vi "Draw Text.vi"(8 "error in (no error)":errorcluster, 11 "Terminal in":refnum<class "Terminal.lvclass">) -> (0 "error out":errorcluster, 3 "Terminal out":refnum<class "Terminal.lvclass">)   [LabVIEW 2020, in "Terminal.lvlib" / "Terminal.lvclass"]
uses:
  Terminal.lvclass
  Text Attributes.ctl
  Terminal.lvclass/Terminal.ctl
  TermBuffer/TermBuffer.lvclass
  Terminal.lvlib
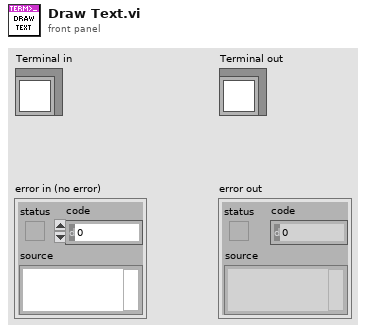
[diagram p1: front panel]
types:
  T1 = cluster{"left":i16, "top":i16, "right":i16, "bottom":i16}
  T2 = enum16{"User-specified Font", "Application Font", "System Font", "Dialog Font"}
  T3 = typedef "Terminal.lvlib/Text Attributes.ctl" = cluster{"FG":u32, "BG":u32, "Bold":bool, "Italic":bool, "Underline":bool, "Strike":bool, "Inverse":bool}
  T4 = typedef "Terminal.lvlib/Terminal.lvclass/Ref Data.ctl" = cluster{"Connection":refnum<class "Connection.lvclass">, "Read Loop Running":bool, "Parse State":T5, "Terminal Options":T9, "Font Metrics":T12}
  T5 = typedef "Terminal.lvlib/Terminal.lvclass/Parse State.ctl" = cluster{"Buffer State":T6, "Cursor":T7, "Attributes":T3}
  T6 = typedef "Terminal.lvlib/Terminal.lvclass/Buffer State.ctl" = cluster{"Sequence":string, "ESC":bool, "Alt Buf":bool}
  T7 = typedef "Terminal.lvlib/Terminal.lvclass/Cursor.ctl" = cluster{"Cur":T8, "Saved":T8}
  T8 = typedef "Terminal.lvlib/Terminal.lvclass/Position.ctl" = cluster{"Row":i32, "Col":i32}
  T9 = typedef "Terminal.lvlib/Terminal Options.ctl" = cluster{"Implied CR with LF":bool, "Local Echo":bool, "Tab Width":i32, "Color Scheme":T10, "Default FG":T11, "Default BG":T11, "History Length":i32, "Font Face":string, "Font Size":i16, "Rows":i32, "Cols":i32}
  T10 = typedef "Terminal.lvlib/Color Scheme.ctl" = cluster{"Black":u32, "Red":u32, "Green":u32, "Yellow":u32, "Blue":u32, "Magenta":u32, "Cyan":u32, "White":u32, "Bright Black":u32, "Bright Red":u32, "Bright Green":u32, "Bright Yellow":u32, "Bright Blue":u32, "Bright Magenta":u32, "Bright Cyan":u32, "Bright White":u32}
  T11 = typedef "Terminal.lvlib/Color.ctl" = i8
  T12 = typedef "Terminal.lvlib/Terminal.lvclass/Font Metrics.ctl" = cluster{"Width":i16, "Height":i16}
  T13 = typedef "Terminal.lvlib/Term Char.ctl" = cluster{"Char":string, "Attributes":T3}
  T14 = cluster{"Font Name:":string, "Size":i16, "Strikeout?":bool, "Italic?":bool, "Underline?":bool, "Outline?":bool, "Shadow?":bool, "Bold?":bool}
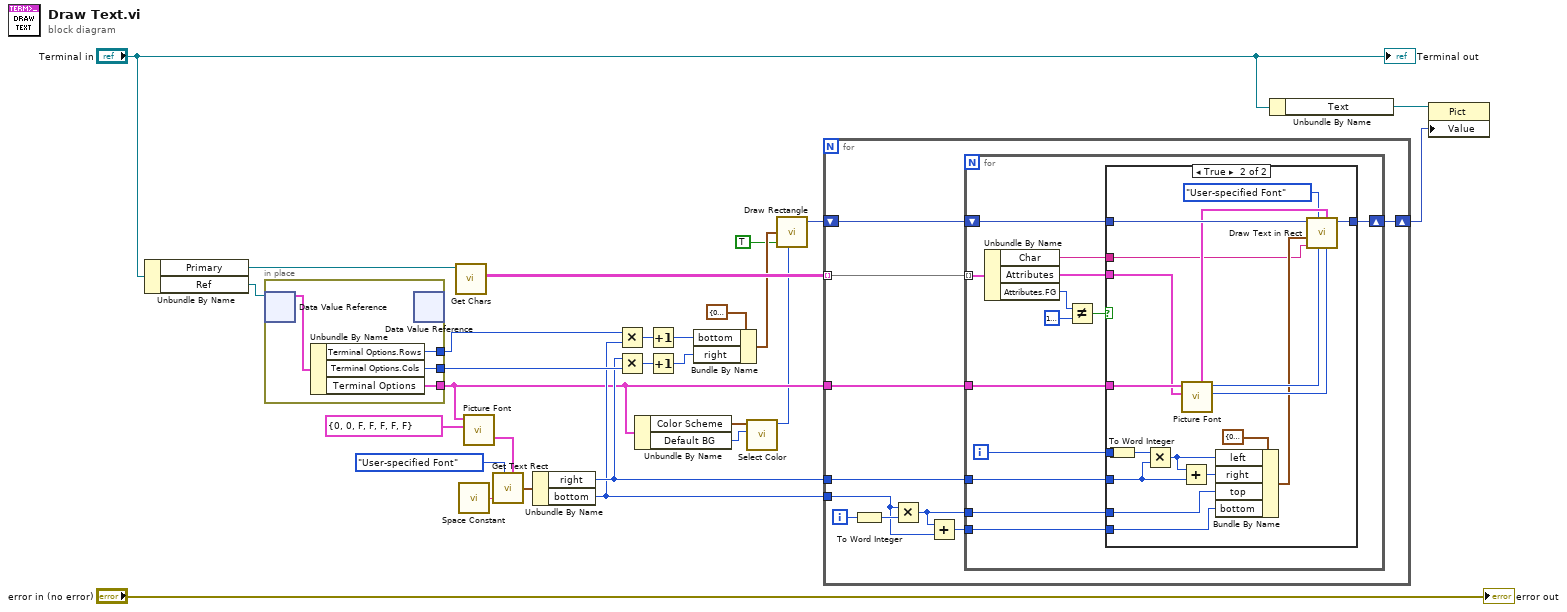
[diagram p0: block diagram]
diagram:
  n1 = Unbundle By Name("Terminal in") -> ("Primary"=w27:refnum<class "TermBuffer.lvclass">, "Ref"=w25:refnum<data-value>)
  n2 = in-place {
    in-place-border: [w31] -> w6
    in-place-border: [w30] -> w13
    in-place-border: [w29] -> w9
    n3 = in-place-dvr #1(w25) -> (w32:T4)  [unwired: 1 out]
    n4 = Unbundle By Name(w32) -> ("Terminal Options.Rows"=w29:i32, "Terminal Options.Cols"=w30:i32, "Terminal Options"=w31:T9)
    n5 = in-place-dvr #1() -> ()  [unwired: 1 in, 2 out]
  }
  n6 = call "Get Chars.vi"("TermBuffer in"=w27) -> ("TermChars"=w26:T13[][])  [unwired: 8 in, 2 out]
  n7 = call <vilib>:"Space Constant.vi"() -> ("String"=w17:string)
  n8 = call "Picture Font.vi"("Text Attributes"=T3 {"FG"=0, "BG"=0, "Bold"=FALSE, "Italic"=FALSE, "Underline"=FALSE, "Strike"=FALSE, "Inverse"=FALSE}, "Terminal Options"=w6) -> ("Picture Font"=w22:T14)  [unwired: 7 in, 2 out]
  n9 = call <vilib>:"Get Text Rect.vi"("desired font(Application)"=T2."User-specified Font", "text"=w17, "[user-specified font]"=w22) -> ("rect"=w21:T1)  [unwired: 6 in]
  n10 = Unbundle By Name(w21) -> ("right"=w12:i16, "bottom"=w10:i16)
  n11 = Multiply(x=w9, y=w10) -> (x*y=w8:i32)
  n12 = Multiply(x=w12, y=w13) -> (x*y=w11:i32)
  n13 = Unbundle By Name(w6) -> ("Color Scheme"=w5:T10, "Default BG"=w4:T11)
  n14 = Increment(x=w8) -> (x+1=w1:i32)
  n15 = Increment(x=w11) -> (x+1=w2:i32)
  n16 = Bundle By Name(cluster=T1 {"left"=0, "top"=0, "right"=0, "bottom"=0} ("rect"), "bottom"=w1, "right"=w2) -> (w14:T1)
  n17 = call "Select Color.vi"("Color"=w4, "Color Scheme"=w5) -> ("Color Value"=w3:u32)  [unwired: 9 in]
  n18 = call <vilib>:"Draw Rectangle.vi"("rect"=w14, "fill?(F)"=TRUE, "color(black)"=w3) -> ("new picture"=w16:picture)  [unwired: 6 in]
  n19 = for {
    tunnel: w26 -> [w42] mode=indexing
    tunnel: w12 -> [w41]
    tunnel: w10 -> [w34]
    shift-right: [w39] -> w18
    shift-left: w16 -> [w40]
    tunnel: w6 -> [w38]
    i -> [w37]
    n20 = To Word Integer(number=w37) -> (16bit integer=w36:i16)
    n21 = Multiply(x=w34, y=w36) -> (x*y=w35:i16)
    n22 = Add(x=w35, y=w34) -> (x+y=w33:i16)
    n23 = for {
      tunnel: w42 -> [w53] mode=indexing
      tunnel: w41 -> [w47]
      shift-right: [w54] -> w39
      shift-left: w40 -> [w55]
      tunnel: w38 -> [w52]
      tunnel: w35 -> [w49]
      tunnel: w33 -> [w48]
      i -> [w50]
      n24 = Unbundle By Name(w53) -> ("Char"=w46:string, "Attributes"=w51:T3, "Attributes.FG"=w45:u32)
      n25 = Not Equal?(x=w45, y=u32 16777216 ("BG")) -> (x != y?=w43:bool)
      n26 = case shown="True" w43 {
        tunnel: w55 -> [w56 w74]
        tunnel: [w56 w73] -> w54
        tunnel: w52 -> [_ w72]
        tunnel: w51 -> [_ w71]
        tunnel: w50 -> [_ w66]
        tunnel: w49 -> [_ w63]
        tunnel: w48 -> [_ w62]
        tunnel: w47 -> [_ w60]
        tunnel: w46 -> [_ w57]
        frame False {
          # "Don't need to draw unset chars"
        }
        frame True {
          n27 = To Word Integer(number=w66) -> (16bit integer=w61:i16)
          n28 = Multiply(x=w61, y=w60) -> (x*y=w58:i16)
          n29 = Add(x=w58, y=w60) -> (x+y=w59:i16)
          n30 = call "Picture Font.vi"("Text Attributes"=w71, "Terminal Options"=w72) -> ("BG"=w67:u32, "FG"=w68:u32, "Picture Font"=w70:T14)  [unwired: 7 in]
          n31 = Bundle By Name(cluster=T1 {"left"=0, "top"=0, "right"=0, "bottom"=0} ("rect"), "left"=w58, "right"=w59, "top"=w63, "bottom"=w62) -> (w64:T1)
          n32 = call <vilib>:"Draw Text in Rect.vi"("BG color(transparent)"=w67, "[user-specified font]"=w70, "text color(black)"=w68, "desired font(Application)"=T2."User-specified Font", "text"=w57, "rect"=w64, "picture"=w74) -> ("new picture"=w73:picture)  [unwired: 4 in]
        }
      }
    }
  }
  n33 = Unbundle By Name("Terminal in") -> ("Text"=w19:refnum<vi>)
  n34 = property class="Pict"(reference=w19, "Value"=w18) -> ()  [unwired: 1 in, 2 out]
  "error out" <- "error in (no error)"
  "Terminal out" <- "Terminal in"
